vi "Add.vi"(8 "error in (no error)":errorcluster, 9 "Value":string, 10 "Key":string, 11 "LUT in":refnum<class "LUT.lvclass">) -> (0 "error out":errorcluster, 3 "LUT out":refnum<class "LUT.lvclass">)   [LabVIEW 2016, in "LUT.lvclass"]
uses:
  LUT.lvclass
  LUT.lvclass/LUT.ctl
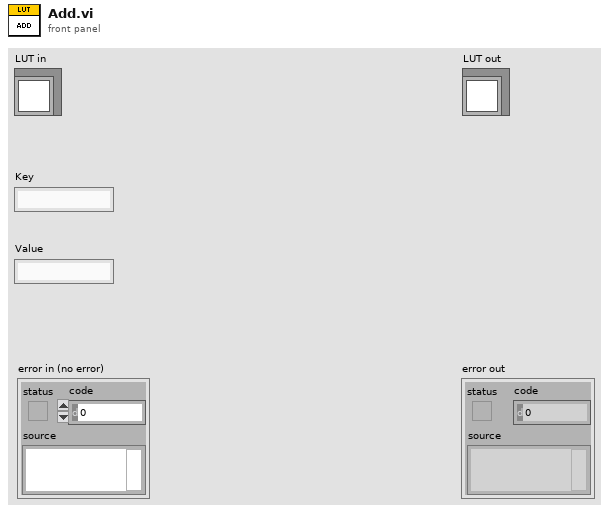
[diagram p1: front panel]
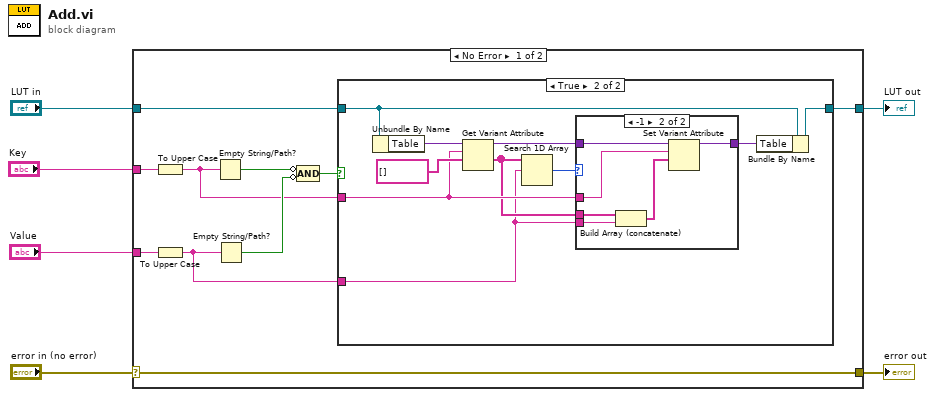
[diagram p0: block diagram]
diagram:
  n1 = case shown="No Error" "error in (no error)" {
    selector: "error in (no error)" -> [w16 w36]
    tunnel: [w16 w36] -> w5
    tunnel: [w7 w35] -> w3
    tunnel: "LUT in" -> [w10 w35]
    tunnel: "Key" -> [w9 _]
    tunnel: "Value" -> [w8 _]
    frame No Error {
      n2 = To Upper Case(1:w9) -> (0:w12:string)
      n3 = To Upper Case(1:w8) -> (0:w11:string)
      n4 = Empty String/Path?(string/path=w12) -> (empty?=w15:bool)
      n5 = Empty String/Path?(string/path=w11) -> (empty?=w14:bool)
      n6 = Compound Arithmetic op=AND(invert w15, invert w14) -> (w13:bool)
      n7 = case shown="True" w13 {
        tunnel: w10 -> [w17 w20]
        tunnel: w12 -> [_ w23]
        tunnel: w11 -> [_ w21]
        tunnel: [w17 w18] -> w7
        frame False {
        }
        frame True {
          n8 = Unbundle By Name(w20) -> ("Table"=w26:variant)
          n9 = Get Variant Attribute(Variant=w26, name=w23, default value (empty Variant)=string[] []) -> (duplicate Variant=w24:variant, value=w22:string[])  [unwired: 1 in, 2 out]
          n10 = Search 1D Array(1D array=w22, element=w21) -> (index of element=w25:i32)  [unwired: 1 in]
          n11 = case shown="-1" w25 {
            tunnel: w24 -> [w28 w34]
            tunnel: w23 -> [_ w33]
            tunnel: w22 -> [_ w32]
            tunnel: w21 -> [_ w31]
            tunnel: [w28 w29] -> w19
            frame Default {
            }
            frame -1 {
              n12 = Build Array (concatenate)(w32, w31) -> (w30:string[])
              n13 = Set Variant Attribute(Variant=w34, name=w33, value=w30) -> (Variant out=w29:variant)  [unwired: 1 in, 2 out]
            }
          }
          n14 = Bundle By Name(cluster=w20, "Table"=w19) -> (w18:refnum<class "LUT.lvclass">)
        }
      }
    }
    frame Error {
    }
  }
  "error out" <- w5
  "LUT out" <- w3
